vi "Colormap from tuple array.vi"(11 "Colormap Elements":cluster{"R":dbl, "G":dbl, "B":dbl, "A":dbl}[](array[cluster])) -> (2 "Value String":string, 3 "Boolean":bool)   [LabVIEW 2021]
uses:
  <vilib>/picture/picture.llb/imagedata.ctl
panel:
  in  "Transpose":bool
  out "new picture":picture
  out "Array":u32[](array[colorbox])
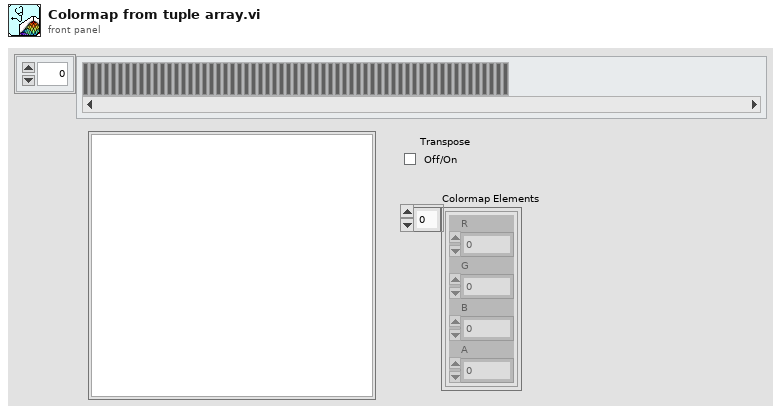
[diagram p1: front panel]
types:
  T1 = typedef "imagedata.ctl" = cluster{"image type":i32, "image depth":i32, "image":u8[], "mask":u8[], "colors":u32[], "Rectangle":cluster{"left":i16, "top":i16, "right":i16, "bottom":i16}}
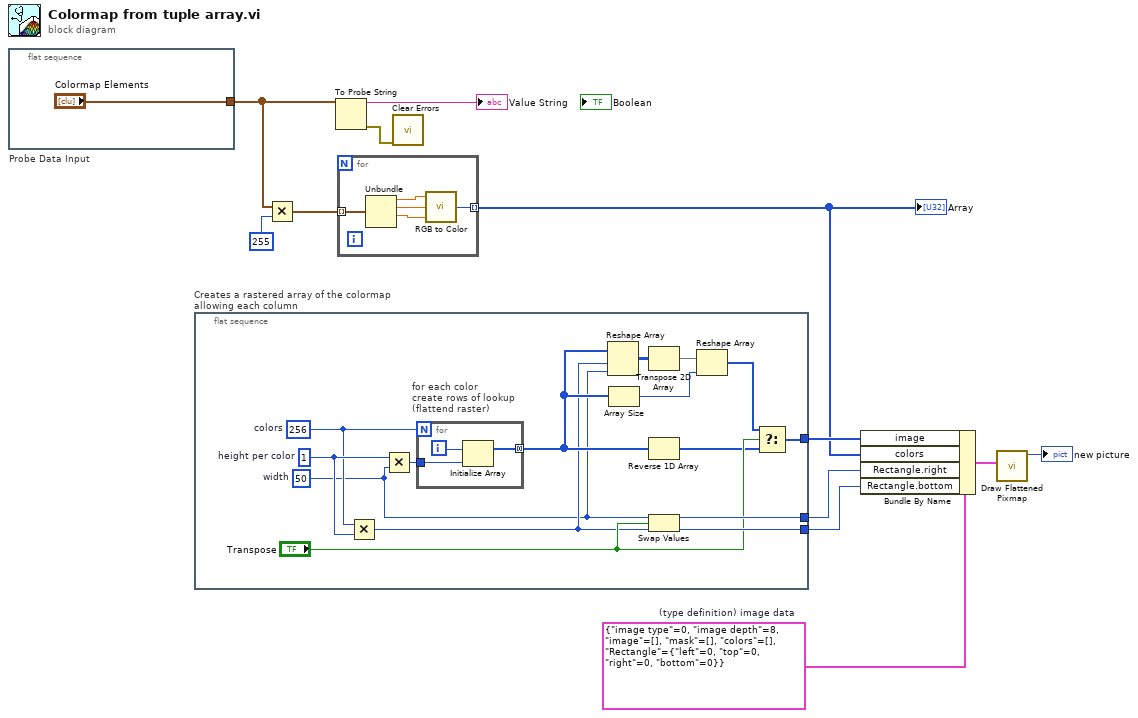
[diagram p0: block diagram]
diagram:
  w10 = T1 {"image type"=0, "image depth"=8, "image"=[], "mask"=[], "colors"=[], "Rectangle"={"left"=0, "top"=0, "right"=0, "bottom"=0}}  # (type definition) image data
  n1 = flat-sequence "Probe Data Input" {
    tunnel: ["Colormap Elements"] -> w11
    frame #0 {
    }
  }
  n2 = flat-sequence "Creates a rastered array of the colormap allowing each column" {
    tunnel: [w24] -> w7
    tunnel: [w23] -> w4
    tunnel: [w22] -> w2
    frame #0 {
      w25 = 256  # colors
      w27 = 1  # height per color
      w16 = 50  # width
      n3 = Multiply(x=w25, y=w27) -> (x*y=w20:i32)
      n4 = Multiply(x=w27, y=w16) -> (x*y=w26:i32)
      n5 = for "for each color\ncreate rows of lookup\n(flattend raster)" {
        N: w25 -> [_]
        tunnel: [w31] -> w28 mode=concatenating
        tunnel: w26 -> [w29]
        i -> [w30]
        n6 = Initialize Array(w30, w29) -> (w31:i32[])
      }
      n7 = Reshape Array(w28, w20, w16) -> (w19:i32[][])
      n8 = Array Size(array=w28) -> (size(s)=w17:i32)
      n9 = Transpose 2D Array(2D array=w19) -> (transposed array=w18:i32[][])
      n10 = Reverse 1D Array(array=w28) -> (reversed array=w14:i32[])
      n11 = Swap Values(12:w16, 13:"Transpose", 14:w20) -> (1:w22:i32, 3:w23:i32)
      n12 = Reshape Array(w18, w17) -> (w15:i32[])
      n13 = Select(t=w15, s="Transpose", f=w14) -> (s? t:f=w24:i32[])
    }
  }
  n14 = Multiply(x=w11, y=u16 255 ("pixels per color")) -> (x*y=w9:cluster{"R":dbl, "G":dbl, "B":dbl, "A":dbl}[])
  n15 = To Probe String(7:w11) -> (0:w1:errorcluster, 3:→"Value String":string)  [unwired: 2 in]
  n16 = for {
    tunnel: w9 -> [w36] mode=indexing
    tunnel: [w32] -> w6 mode=indexing
    n17 = Unbundle(w36) -> ("R"=w35:dbl, "G"=w34:dbl, "B"=w33:dbl)  [unwired: 1 out]
    n18 = call <vilib>:"RGB to Color.vi"("B"=w33, "G"=w34, "R"=w35) -> ("Color"=w32:u32)
  }
  "Array" <- w6
  n19 = call <vilib>:"Clear Errors.vi"("error in (no error)"=w1) -> ()  [unwired: 5 in, 2 out]
  n20 = Bundle By Name(cluster=w10, "image"=w7, "colors"=w6, "Rectangle.right"=w2, "Rectangle.bottom"=w4) -> (w8:T1)
  n21 = call <vilib>:"Draw Flattened Pixmap.vi"("image data"=w8) -> ("new picture"=→"new picture":picture)  [unwired: 8 in]
